vi "Flow Global.vi"() -> ()   [LabVIEW 2018]
panel:
  in  "Flow Hz 2":dbl
  in  "Current Tolerance":dbl
  in  "Flow Hz":dbl
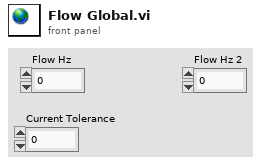
[diagram p1: front panel]
diagram:
